vi "take_photo.vi"() -> ()   [LabVIEW 2019]
uses:
  <vilib>/vision/Image Controls.llb/IMAQ Image.ctl
  <vilib>/userdefined/High Color/IMAQdx.ctl
  <vilib>/vision/driver/IMAQdx.llb/IMAQdx Buffer Number Mode.ctl
  <vilib>/vision/driver/NI_Vision_Acquisition_Software.lvlib
panel:
  out "identifying number":string
  out "Queue":string
  in  "Image":T1
  in  "stop":bool
  in  "take a photo":bool
  out "实时":T1(plugin-control)
  in  "save":bool
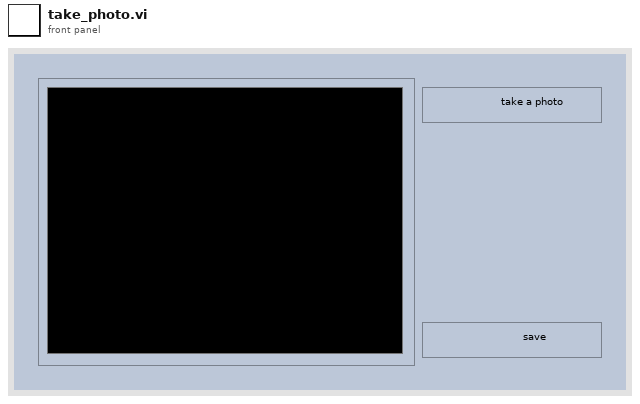
[diagram p1: front panel]
types:
  T1 = typedef "IMAQ Image.ctl" = refnum<image>
  T2 = typedef "IMAQdx.ctl" = refnum<k21>
  T3 = typedef "NI_Vision_Acquisition_Software.lvlib/IMAQdx Buffer Number Mode.ctl" = enum32{"Next", "Last", "Buffer Number", "Every", "Last New"}
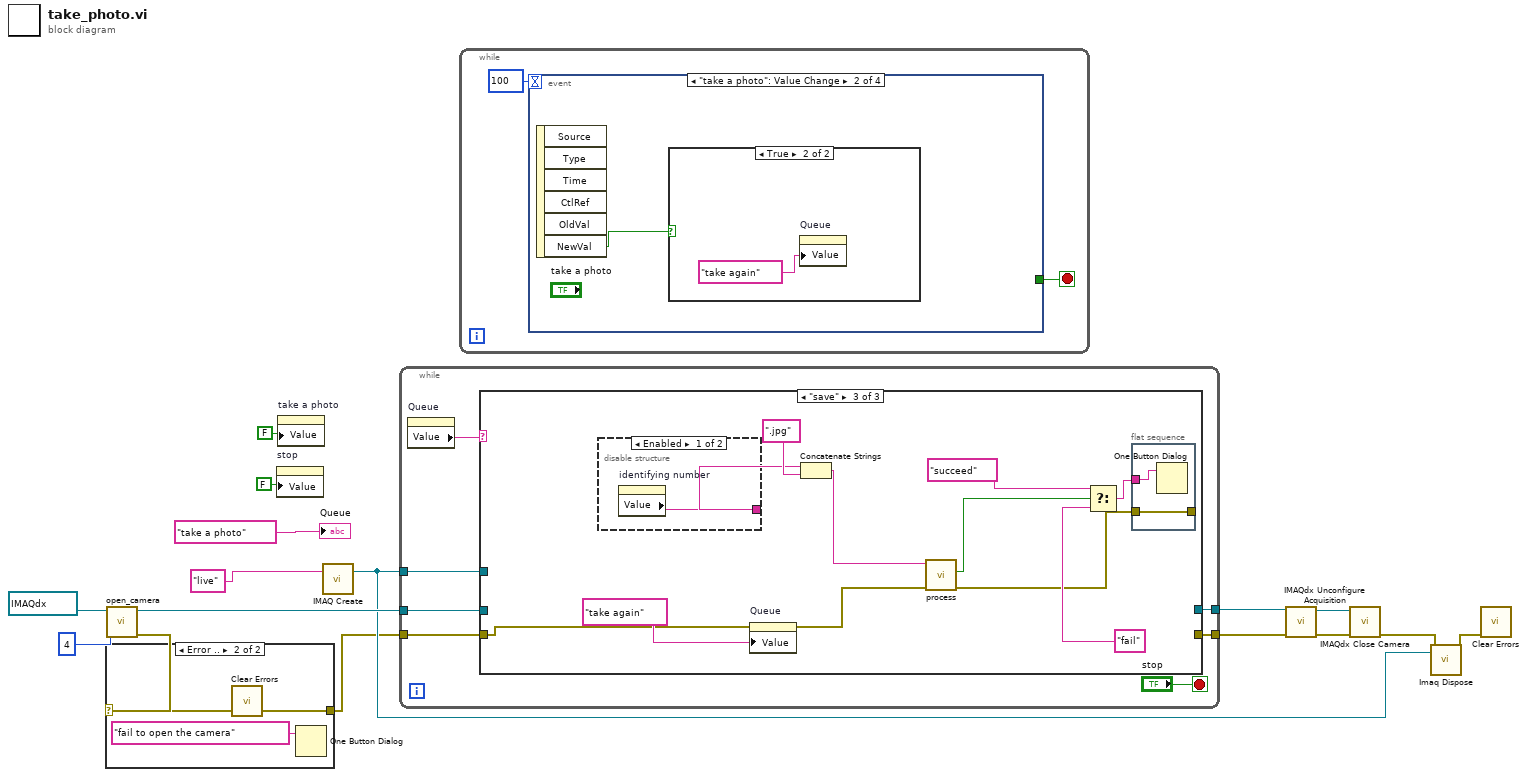
[diagram p0: block diagram]
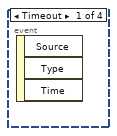
[diagram p3: hidden frame]
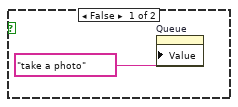
[diagram p4: hidden frame]
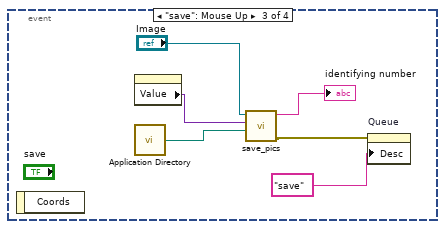
[diagram p5: hidden frame]
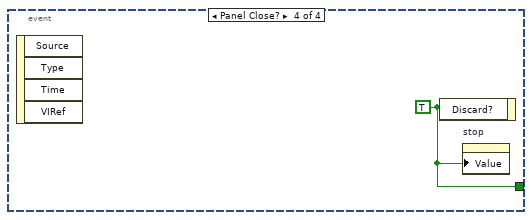
[diagram p6: hidden frame]
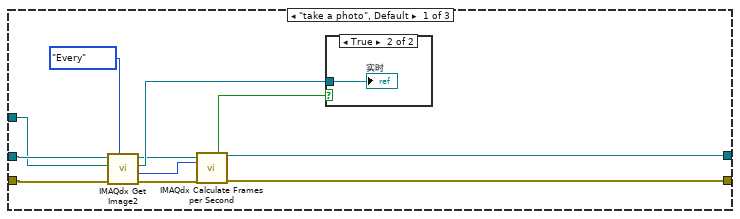
[diagram p7: hidden frame]
diagram:
  n1 = call "open_camera.vi"("VideoMode"=u32 4, "Session In"=T2 "cam0") -> ("error out"=w6:errorcluster, "Session Out"=w12:T2)  [unwired: 8 in]
  n2 = case shown="Error .." w6 {
    selector: w6 -> [w17 w20]
    tunnel: [w17 w19] -> w5
    frame No Error {
    }
    frame Error {
      n3 = call <vilib>:"Clear Errors.vi"("error in (no error)"=w20) -> ("error out"=w19:errorcluster)  [unwired: 5 in, 1 out]
      n4 = One Button Dialog(message="fail to open the camera") -> ()  [unwired: 1 in, 1 out]
    }
  }
  n5 = property on="stop" class="Bool (strict)"("Value"=FALSE ("停止")) -> ()  [unwired: 2 in, 2 out]
  n6 = property on="take a photo" class="Bool (strict)"("Value"=FALSE ("拍照按钮")) -> ()  [unwired: 2 in, 2 out]
  n7 = call "IMAQ Create"("Image Name"="live") -> ("New Image"=w11:T1)  [unwired: 4 in, 1 out]
  n8 = while {
    tunnel: w12 -> [w27]
    tunnel: w5 -> [w26]
    tunnel: w11 -> [w25]
    tunnel: [w24] -> w13
    tunnel: [w23] -> w2
    stop <- "stop" stop-if-true
    n9 = property on="Queue" class="Str"() -> ("Value"=w21:string)  [unwired: 2 in, 2 out]
    n10 = case shown="\"save\"" w21 {
      tunnel: w27 -> [w32 _ _]
      tunnel: w26 -> [w31 _ w42]
      tunnel: w25 -> [w30 _ _]
      tunnel: [w29 _ _] -> w24
      tunnel: [w28 _ _] -> w23
      frame "take a photo", Default {
        n11 = call <vilib>:"IMAQdx Get Image2.vi"("Buffer Number Mode (Next)"=IMAQdx_Buffer_Number_Mode."Every", "error in"=w31, "Image In"=w30, "Session In"=w32) -> ("error out"=w34:errorcluster, "Buffer Number Out"=w36:u32, "Image Out"=w38:T1, "Session Out"=w33:T2)  [unwired: 4 in]
        n12 = call <vilib>:"IMAQdx Calculate Frames per Second.vi"("Session In"=w33, "Buffer Number"=w36, "error in (no error)"=w34) -> ("Update Display"=w37:bool, "Session Out"=w29:T2, "error out"=w28:errorcluster)  [unwired: 6 in, 4 out]
        n13 = case shown="True" w37 {
          tunnel: w38 -> [_ w39]
          frame False {
          }
          frame True {
            "实时" <- w39
          }
        }
      }
      frame "take again" {
      }
      frame "save" {
        n14 = disable-structure shown="Enabled" {
          disable-tunnel: [w51 w52] -> w43
          frame Enabled {
            n15 = property on="identifying number" class="Str"() -> ("Value"=w51:string)  [unwired: 2 in, 2 out]
          }
          frame Disabled {
          }
        }
        n16 = property on="Queue" class="Str"(error in=w42, "Value"="take again" ("字符串")) -> (error out=w41:errorcluster)  [unwired: 1 in, 1 out]
        n17 = Concatenate Strings(w43, ".jpg" ("字符串")) -> (w49:string)
        n18 = call "process.vi"("error in (no error)"=w41, "img_name"=w49) -> ("error out"=w45:errorcluster, "返回值"=w40:bool)  [unwired: 8 in]
        n19 = Select(t="succeed" ("字符串"), s=w40, f="fail" ("字符串")) -> (s? t:f=w46:string)
        n20 = flat-sequence {
          tunnel: w46 -> [w54]
          tunnel: w45 -> [w53]
          tunnel: [w53] -> _
          frame #0 {
            n21 = One Button Dialog(message=w54) -> ()  [unwired: 1 in, 1 out]
          }
        }
      }
    }
  }
  n22 = while {
    stop <- w55 stop-if-true
    n23 = event shown="[1] \"take a photo\": Value Change" {
      selector: _ -> [_ _ _ _]
      dyn-events: _ -> [_ _ _ _]
      timeout: 100 -> [_ _ _ _]
      tunnel: [_ _ _ w66] -> w55
      event Timeout {
        n24 = event-data() -> ()  [unwired: 1 in, 3 out]
      }
      event "take a photo": Value Change {
        n25 = event-data() -> ("NewVal"=w57:bool)  [unwired: 1 in, 5 out]
        n26 = case shown="True" w57 {
          frame False {
            n27 = property on="Queue" class="Str"("Value"="take a photo" ("队列")) -> ()  [unwired: 2 in, 2 out]
          }
          frame True {
            n28 = property on="Queue" class="Str"("Value"="take again" ("队列")) -> ()  [unwired: 2 in, 2 out]
          }
        }
      }
      event "save": Mouse Up {
        n29 = event-data() -> ()  [unwired: 1 in, 1 out]
        n30 = property on="实时" class="ImageControl"() -> ("Value"=w60:variant)  [unwired: 2 in, 2 out]
        n31 = call <vilib>:"Application Directory.vi"() -> ("Application Directory"=w63:path)
        n32 = call "save_pics.vi"("path"=w63, "变体"=w60, "IMAQ image.ctl"="Image") -> ("error out"=w64:errorcluster, "identifying number"=→"identifying number":string)  [unwired: 7 in]
        n33 = property on="Queue" class="Str"(error in=w64, "Desc"="save" ("队列")) -> ()  [unwired: 1 in, 2 out]
      }
      event Panel Close? {
        w66 = TRUE ("放弃？")
        n34 = event-data() -> ()  [unwired: 1 in, 4 out]
        n35 = event-data("Discard?"=w66) -> ()  [unwired: 1 in, 1 out]
        n36 = property on="stop" class="Bool (strict)"("Value"=w66) -> ()  [unwired: 2 in, 2 out]
      }
    }
  }
  n37 = call <vilib>:"IMAQdx Unconfigure Acquisition.vi"("error in"=w2, "Session In"=w13) -> ("error out"=w15:errorcluster, "Session Out"=w16:T2)  [unwired: 8 in]
  n38 = call <vilib>:"IMAQdx Close Camera.vi"("error in"=w15, "Session In"=w16) -> ("error out"=w14:errorcluster)  [unwired: 9 in]
  n39 = call "Imaq Dispose"("Image"=w11, "error in (no error)"=w14) -> ("error out"=w4:errorcluster)  [unwired: 4 in]
  n40 = call <vilib>:"Clear Errors.vi"("error in (no error)"=w4) -> ()  [unwired: 5 in, 2 out]
  "Queue" <- "take a photo" ("队列")
